vi "GetDocStrings.vi"(6 "error in":errorcluster, 9 "path in":path) -> (0 "error out":errorcluster, 3 "path out":path, 4 "docstrings":T1[](array[typedef]), 5 "short name":string)   [LabVIEW 2014, in "Raspberry Pi Compatible Compiler for LabVIEW.lvlib" / "Python Functions.lvlib"]
uses:
  Python Functions.lvlib
  DocstringTD.ctl
  <vilib>/regexp/Match Regular Expression.xnode
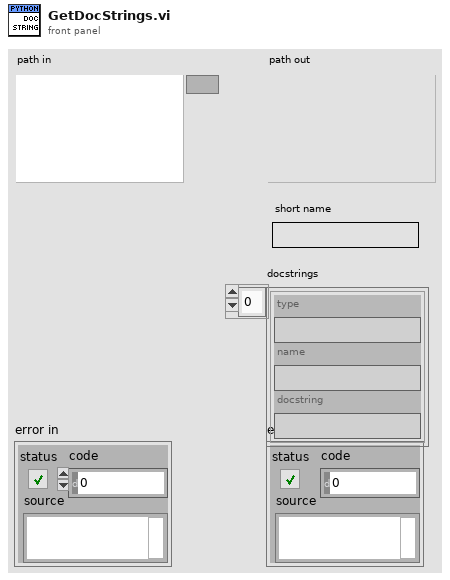
[diagram p1: front panel]
types:
  T1 = typedef "Raspberry Pi Compatible Compiler for LabVIEW.lvlib/Python Functions.lvlib/DocstringTD.ctl" = cluster{"type":string, "name":string, "docstring":string}
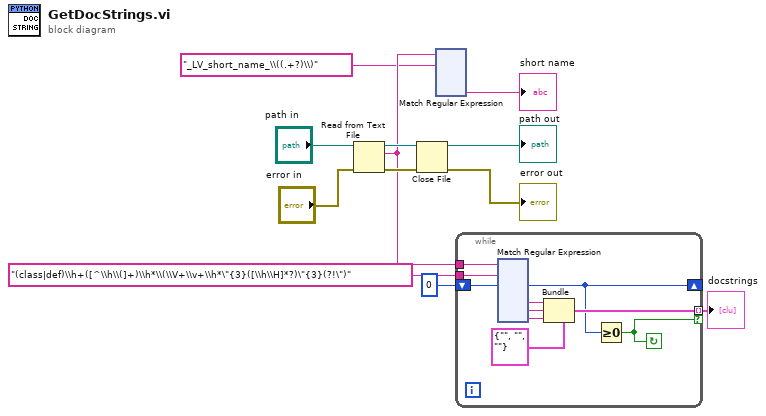
[diagram p0: block diagram]
diagram:
  n1 = Read from Text File(file (use dialog)="path in", error in="error in") -> (refnum out=w9:refnum<file>, text=w3:string, error out=w10:errorcluster)  [unwired: 2 in, 1 out]
  n2 = Close File(refnum=w9, error in=w10) -> (path=→"path out":path, error out=→"error out":errorcluster)
  n3 = xnode "Match Regular Expression"("input string"=w3, "regular expression"="_LV_short_name_\\((.+?)\\)") -> ("submatch 1"=→"short name":string)  [unwired: 4 in, 5 out]
  n4 = while {
    shift-right: [w14] -> _
    shift-left: 0 -> [w21]
    tunnel: w3 -> [w22]
    tunnel: "(class|def)\\h+([^\\h\\(]+)\\h*\\(\\V+\\v+\\h*\"{3}([\\h\\H]*?)\"{3}(?!\")" ("regular expression") -> [w20]
    tunnel: [w15] -> w4 mode=indexing if=w13
    stop <- w13 continue-if-true
    n5 = xnode "Match Regular Expression"("input string"=w22, "regular expression"=w20, "offset (0)"=w21) -> ("offset past match"=w14:i32, "submatch 1"=w19:string, "submatch 2"=w17:string, "submatch 3"=w16:string)  [unwired: 3 in, 4 out]
    n6 = Bundle(cluster=T1 {"type"="", "name"="", "docstring"=""} ("docstrings"), "type"=w19, "name"=w17, "docstring"=w16) -> (w15:T1)
    n7 = Greater Or Equal To 0?(x=w14) -> (x >= 0?=w13:bool)
  }
  "docstrings" <- w4
